vi "JKI pwd controller.vi"(0 "Titlebar Text (\"\")":string, 5 "Status Text (\"\")":string, 7 "Animation (3)":u16(ring)=3, 11 "error in (no error)":errorcluster, 12 "Action (Update Message)":T1=enum."Update Message") -> (15 "error out":errorcluster)   [LabVIEW 2012]
doc: "Thus is the main VI that is used to controll the please wait dialog.\n\n<B>Action:</B> This has the following options:\nTurn On: This should be set first. In this mode you can also pass text for the initial status message, titlebar text and the preffered animation.\nTurn Off: Run this mode to turn off (close) the dialog.\nUpdate Message: Run this mode to update the message when the dialog is already running.\n\n<B>Titlebar Text:</B> This is the text you want to display in the titlebar of the dialog. This can only be set during the \"turn on\" action, upon launch.\n\n<B>Status Text:</B> This is the text to display in the center of the dialog.\n\n<B>Animation:</B> This is the index of the built-in animations available for the dialog. Setting this value to 0 will disable the animation. This can only be set during the \"turn on\" action, upon launch. The status text is still available in this mode.\n\nJKI Please Wait Dialog V1.0.2\nCopyright © 2006, James Kring, Inc.\nAll rights reserved.\n\nAuthor:\nMichael Aivaliotis\n<email: michael.aivaliotis@jameskring.com>\n<alternate email: michael@aivaliotis.com>"
uses:
  support/controls/JKI pwd controller action.ctl
  support/controls/JKI pwd queue manager mode enum.ctl
panel:
  # "JKI Please Wait Dialog V1.0.2\nCopyright © 2006, James Kring, Inc.\nAll rights reserved.\n\nAuthor:\nMichael Aivaliotis\n<email: michael.aivaliotis@jameskring.com>\n<alternate email: michael@aivaliotis.com>"
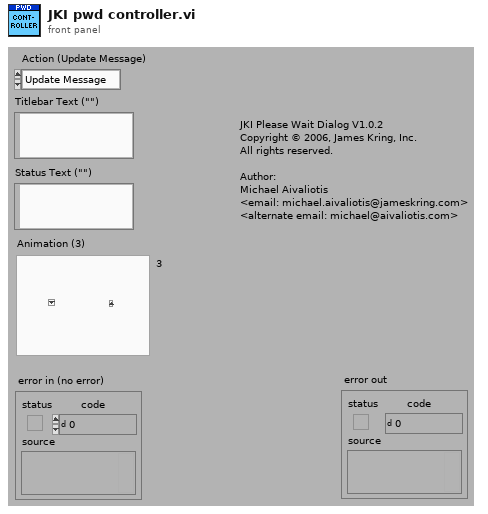
[diagram p1: front panel]
types:
  T1 = typedef "JKI pwd controller action.ctl" = enum16{"Turn On", "Turn Off", "Update Message"}
  T2 = typedef "JKI pwd queue manager mode enum.ctl" = enum16{"< idle >", "Get Refnum", "Send Message"}
  T3 = enum32{"invalid app kind", "Development System", "Run Time System", "Student Edition", "Embedded LabVIEW", "Evaluation", "Custom"}
  T4 = enum32{"Bad", "Idle", "Run top level", "Running"}
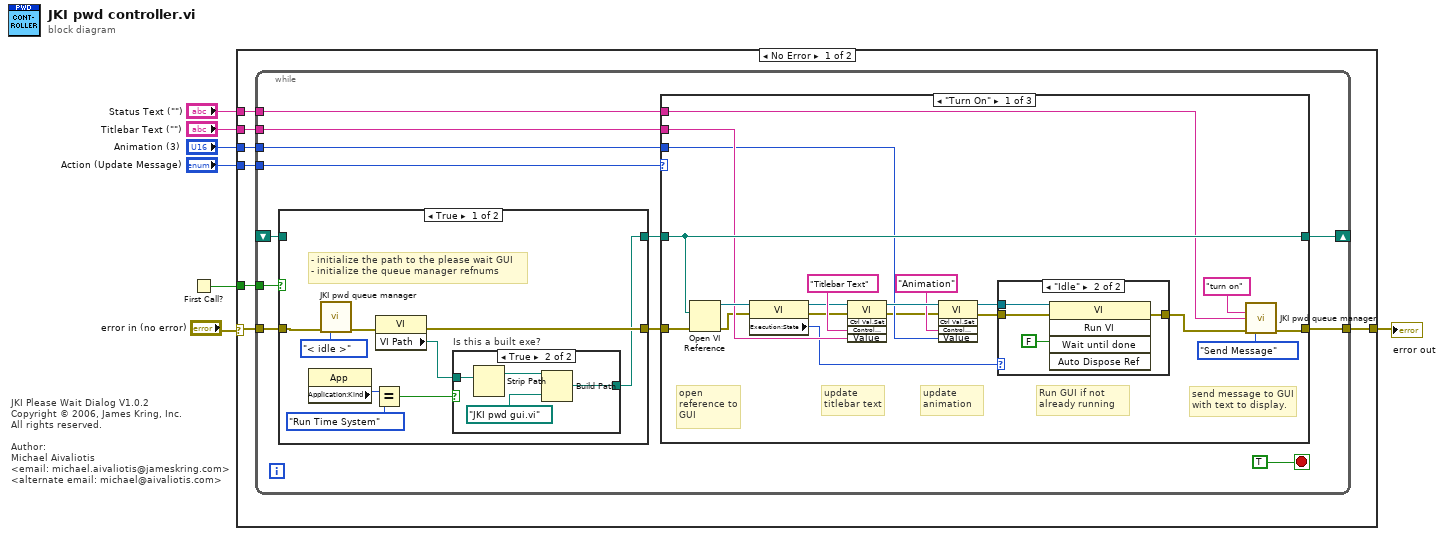
[diagram p0: block diagram]
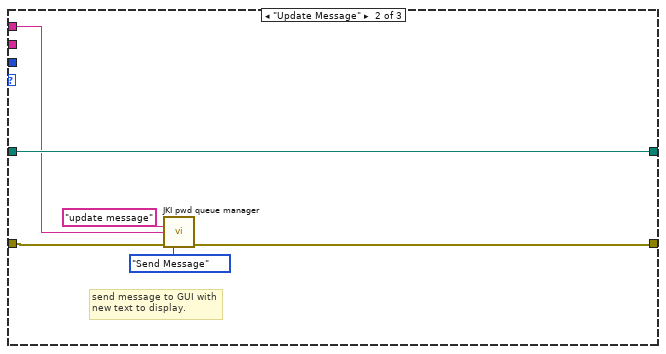
[diagram p3: hidden frame]
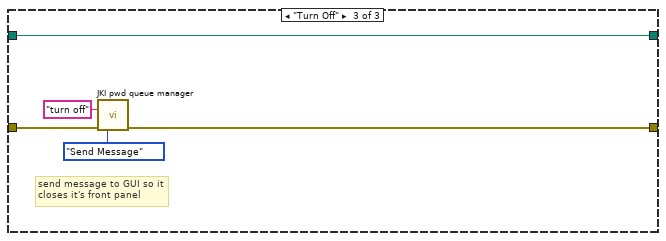
[diagram p4: hidden frame]
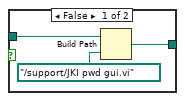
[diagram p5: hidden frame]
diagram:
  # "JKI Please Wait Dialog V1.0.2\nCopyright © 2006, James Kring, Inc.\nAll rights reserved.\n\nAuthor:\nMichael Aivaliotis\n<email: michael.aivaliotis@jameskring.com>\n<alternate email: michael@aivaliotis.com>"
  n1 = First Call?() -> (First Call?: T/F=w7:bool)
  n2 = case shown="No Error" "error in (no error)" {
    selector: "error in (no error)" -> [w9 w81]
    tunnel: w7 -> [w14 _]
    tunnel: "Action (Update Message)" -> [w13 _]
    tunnel: "Titlebar Text (\"\")" -> [w12 _]
    tunnel: "Animation (3)" -> [w11 _]
    tunnel: "Status Text (\"\")" -> [w10 _]
    tunnel: [w8 w81] -> w1
    frame No Error {
      n3 = while {
        shift-right: [w22] -> _
        shift-left: _ -> [w26]
        tunnel: w14 -> [w24]
        tunnel: w13 -> [w21]
        tunnel: w9 -> [w20]
        tunnel: w12 -> [w18]
        tunnel: w11 -> [w17]
        tunnel: w10 -> [w16]
        tunnel: [w15] -> w8
        stop <- TRUE stop-if-true
        n4 = case shown="True" w24 {
          tunnel: w26 -> [_ w80]
          tunnel: [w67 w80] -> w23
          tunnel: [w71 w79] -> w19
          tunnel: w20 -> [w70 w79]
          frame True {
            # "- initialize the path to the please wait GUI\n- initialize the queue manager refnums"
            n5 = property class="App"() -> ("Application:Kind"=w66:T3)  [unwired: 2 in, 2 out]
            n6 = call "JKI pwd queue manager.vi"("error in (no error)"=w70, "Mode (Get Refnum)"=JKI_pwd_queue_manager_mode_enum."< idle >") -> ("error out"=w69:errorcluster)  [unwired: 12 in, 1 out]
            n7 = Equal?(x=w66, y=T3."Run Time System") -> (x = y?=w63:bool)
            n8 = property class="VI"(error in=w69) -> (error out=w71:errorcluster, "VI Path"=w64:path)  [unwired: 1 in, 1 out]
            n9 = case "Is this a built exe?" shown="True" w63 {
              tunnel: [w73 w76] -> w67
              tunnel: w64 -> [w72 w78]
              frame False {
                n10 = Build Path(base path=w72, name or relative path=path "../support/JKI pwd gui.vi") -> (appended path=w73:path)
              }
              frame True {
                n11 = Strip Path(path=w78) -> (stripped path=w77:path)  [unwired: 1 out]
                n12 = Build Path(base path=w77, name or relative path=path "JKI pwd gui.vi") -> (appended path=w76:path)
              }
            }
          }
          frame False {
          }
        }
        n13 = case shown="\"Turn On\"" w21 {
          tunnel: w23 -> [w45 w57 w62]
          tunnel: [w45 w57 w62] -> w22
          tunnel: w19 -> [w46 w53 w59]
          tunnel: w18 -> [w42 _ _]
          tunnel: w17 -> [w39 _ _]
          tunnel: w16 -> [w28 w54 _]
          tunnel: [w31 w52 w58] -> w15
          frame "Turn On" {
            # "send message to GUI with text to display."
            # "Run GUI if not already running"
            # "update animation"
            # "update titlebar text"
            # "open reference to GUI"
            n14 = Open VI Reference(vi path=w45, error in (no error)=w46) -> (vi reference=w44:refnum<vi>, error out=w35:errorcluster)  [unwired: 4 in]
            n15 = property class="VI"(reference=w44, error in=w35) -> (reference out=w34:refnum<vi>, error out=w33:errorcluster, "Execution:State"=w32:T4)
            n16 = invoke class="VI" method="Ctrl Val.Set"(reference=w34, error in=w33, "Control Name"="Titlebar Text", "Value"=w42) -> (reference out=w41:refnum<vi>, error out=w38:errorcluster)  [unwired: 1 in, 3 out]
            n17 = invoke class="VI" method="Ctrl Val.Set"(reference=w41, error in=w38, "Control Name"="Animation", "Value"=w39) -> (reference out=w37:refnum<vi>, error out=w36:errorcluster)  [unwired: 1 in, 3 out]
            n18 = case shown="\"Idle\"" w32 {
              tunnel: w37 -> [_ w51]
              tunnel: w36 -> [w47 w50]
              tunnel: [w47 w49] -> w30
              frame Default {
              }
              frame "Idle" {
                n19 = invoke class="VI" method="Run VI"(reference=w51, error in=w50, "Wait until done"=FALSE) -> (error out=w49:errorcluster)  [unwired: 2 in, 4 out]
              }
            }
            n20 = call "JKI pwd queue manager.vi"("Command (\"\")"="turn on" ("command"), "Variant Data (\"\")"=w28, "error in (no error)"=w30, "Mode (Get Refnum)"=JKI_pwd_queue_manager_mode_enum."Send Message") -> ("error out"=w31:errorcluster)  [unwired: 10 in, 1 out]
          }
          frame "Update Message" {
            # "send message to GUI with new text to display."
            n21 = call "JKI pwd queue manager.vi"("Command (\"\")"="update message" ("Command (\"\")"), "Variant Data (\"\")"=w54, "error in (no error)"=w53, "Mode (Get Refnum)"=JKI_pwd_queue_manager_mode_enum."Send Message") -> ("error out"=w52:errorcluster)  [unwired: 10 in, 1 out]
          }
          frame "Turn Off" {
            # "send message to GUI so it closes it's front panel"
            n22 = call "JKI pwd queue manager.vi"("Command (\"\")"="turn off" ("Command (\"\")"), "error in (no error)"=w59, "Mode (Get Refnum)"=JKI_pwd_queue_manager_mode_enum."Send Message") -> ("error out"=w58:errorcluster)  [unwired: 11 in, 1 out]
          }
        }
      }
    }
    frame Error {
    }
  }
  "error out" <- w1
